vi "Create EPTx Page.vi"(8 "error in (no error)":errorcluster, 11 "Section Ptr":T1 format="%.0x") -> (0 "error out":errorcluster, 3 "Parent Ref out":T1 format="%.0x")   [LabVIEW 2015, in "DCM System Explorer.lvlib"]
uses:
  DCM System Explorer.lvlib
  <vilib>/NI Veristand/Custom Device API/Custom Device Item Ref.ctl
  <vilib>/NI Veristand/Custom Device API/Custom Device Channel Type.ctl
  Shared/DCM Constants and GUIDs.vi
  <vilib>/NI VeriStand/Custom Device API/Custom Device API.lvlib
  DCM Shared.lvlib
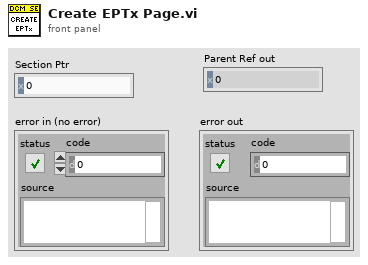
[diagram p1: front panel]
types:
  T1 = typedef "Custom Device API.lvlib/Custom Device Item Ref.ctl" = u64
  T2 = typedef "Custom Device API.lvlib/Custom Device Channel Type.ctl" = enum16{"Input", "Output"}
  T3 = typedef "DCM Shared.lvlib/Channel.ctl" = cluster{"Name":string, "Units":string, "Default":dbl, "Description":string}
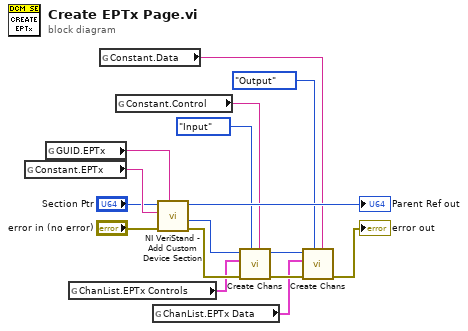
[diagram p0: block diagram]
diagram:
  n1 = global read "DCM Constants and GUIDs.vi" "Constant.EPTx"() -> (w14:string)
  n2 = global read "DCM Constants and GUIDs.vi" "GUID.EPTx"() -> (w15:string)
  n3 = global read "DCM Constants and GUIDs.vi" "ChanList.EPTx Controls"() -> (w8:T3[])
  n4 = global read "DCM Constants and GUIDs.vi" "Constant.Data"() -> (w2:string)
  n5 = global read "DCM Constants and GUIDs.vi" "Constant.Control"() -> (w3:string)
  n6 = global read "DCM Constants and GUIDs.vi" "ChanList.EPTx Data"() -> (w1:T3[])
  n7 = call <vilib>:"NI VeriStand - Add Custom Device Section.vi"("GUID (Default Section)"=w15, "error in (no error)"="error in (no error)", "Section Name"=w14, "Parent Ref in"="Section Ptr") -> ("error out"=w11:errorcluster, "Section Ptr"=w9:T1, "Parent Ref out"=→"Parent Ref out":T1)  [unwired: 4 in, 1 out]
  n8 = call "Create Chans.vi"("New Section Name (none)"=w3, "Type"=Custom_Device_Channel_Type."Input", "error in (no error)"=w11, "Channels"=w8, "Section Ptr"=w9) -> ("error out"=w6:errorcluster, "Section Ptr dup"=w7:T1)  [unwired: 3 in, 2 out]
  n9 = call "Create Chans.vi"("New Section Name (none)"=w2, "Type"=Custom_Device_Channel_Type."Output", "error in (no error)"=w6, "Channels"=w1, "Section Ptr"=w7) -> ("error out"=→"error out":errorcluster)  [unwired: 3 in, 3 out]
